vi "Arduino_Timed_Gate.vi"() -> (5 "Plug in titles":string[](array[string]), 7 "Plug in values":string[](array[string]))   [LabVIEW 2013]
uses:
  Controls/Post_Process.ctl
  Controls/Setup.ctl
  Globals/Meas_global.vi
panel:
  out "Current state":string
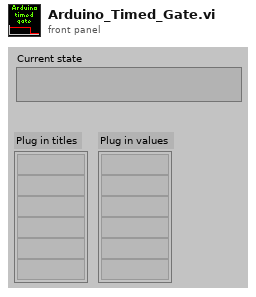
[diagram p1: front panel]
types:
  T1 = typedef "Setup.ctl" = enum16{"Run Program", "Show Setup", "Save Current Setup", "Setup Front Panel"}
  T2 = typedef "Post_Process.ctl" = enum16{"Take New Data", "Post Process Raw Data File"}
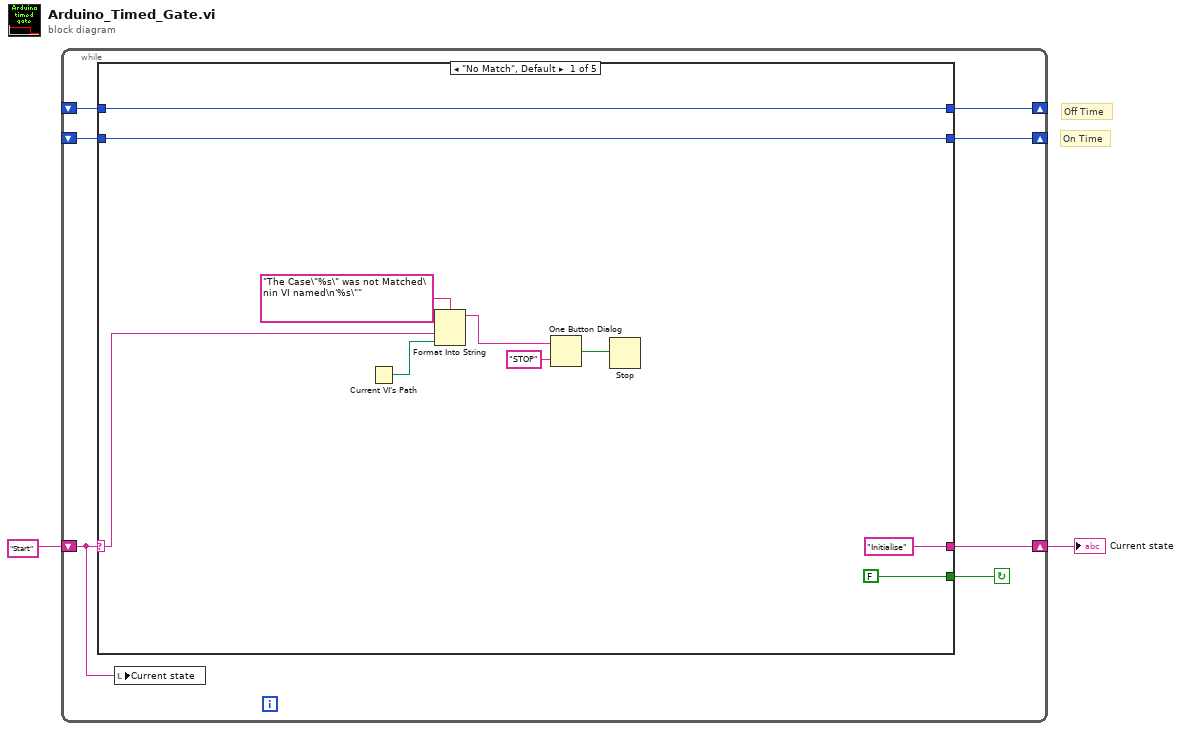
[diagram p0: block diagram]
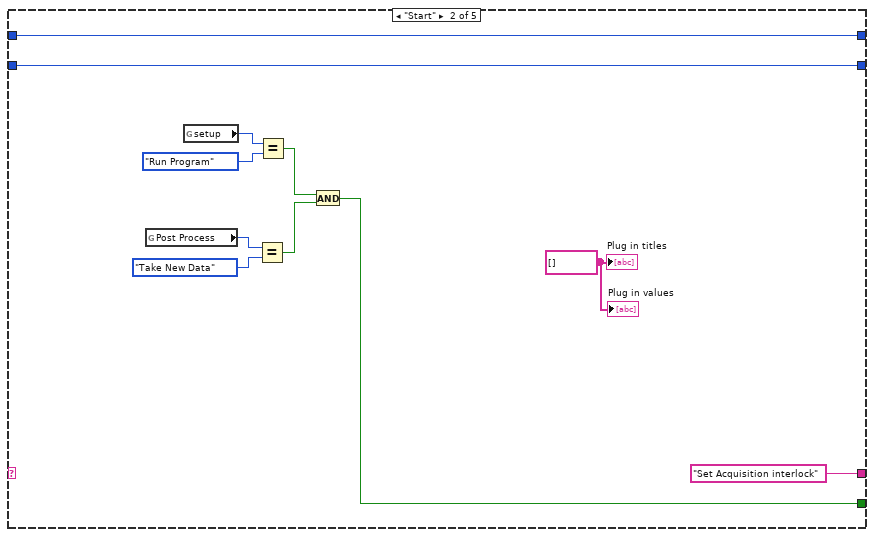
[diagram p2: hidden frame]
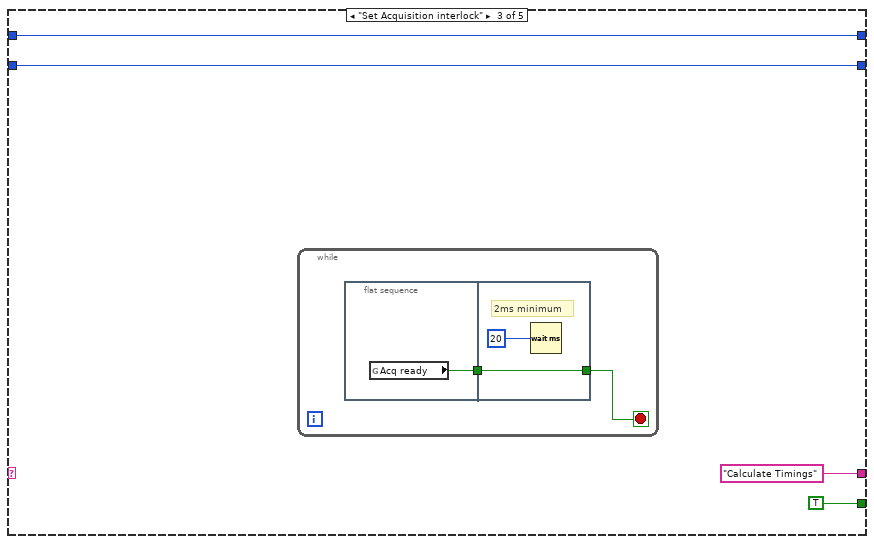
[diagram p3: hidden frame]
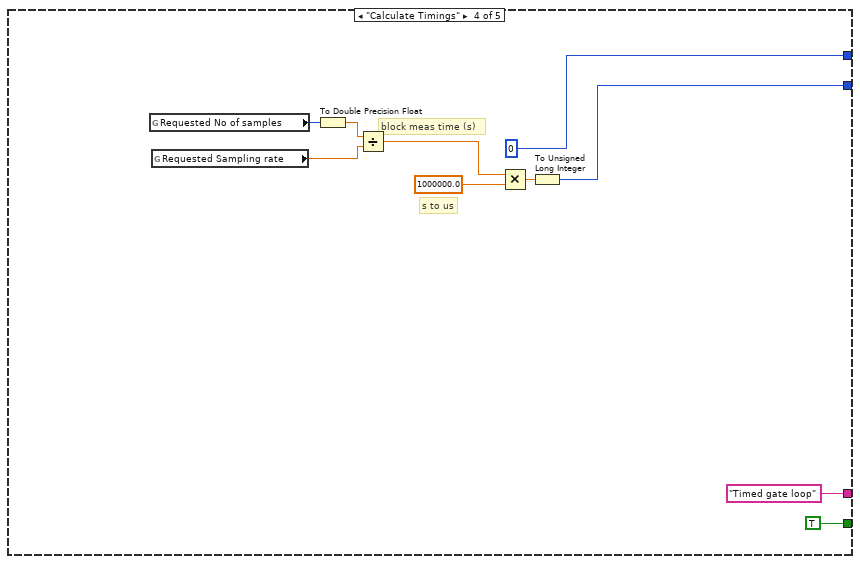
[diagram p4: hidden frame]
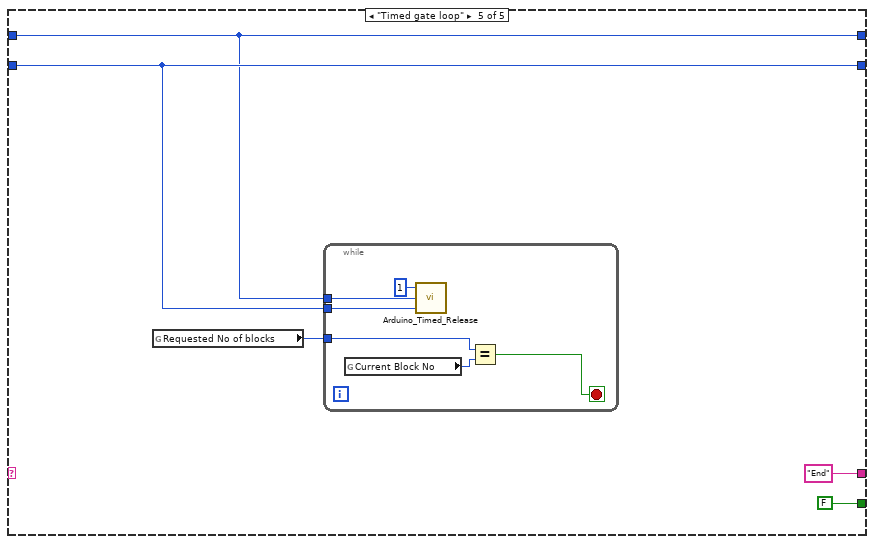
[diagram p5: hidden frame]
diagram:
  # "On Time"
  # "Off Time"
  n1 = while {
    shift-left: "Start" -> [w3]
    shift-right: [w8] -> w1
    shift-right: [w7] -> _
    shift-left: _ -> [w6]
    shift-right: [w5] -> _
    shift-left: _ -> [w4]
    stop <- w9 continue-if-true
    n2 = case shown="\"No Match\", Default" w3 {
      selector: w3 -> [w10 _ _ _ _]
      tunnel: [FALSE w22 TRUE ("Command Found") TRUE ("Command Found") FALSE ("Command Found")] -> w9
      tunnel: ["Initialise" "Set Acquisition interlock" "Calculate Timings" "Timed gate loop" "End"] -> w8
      tunnel: [w12 w21 w32 u32 0 ("number") w51] -> w7
      tunnel: w6 -> [w12 w21 w32 _ w51]
      tunnel: [w11 w20 w31 w44 w54] -> w5
      tunnel: w4 -> [w11 w20 w31 _ w54]
      frame "No Match", Default {
        n3 = Current VI's Path() -> (path=w14:path)
        n4 = Format Into String(format string="The Case\"%s\" was not Matched\nin VI named\n'%s\"" ("Format String"), w10, w14) -> (resulting string=w17:string)  [unwired: 2 in, 1 out]
        n5 = One Button Dialog(message=w17, button name ("OK")="STOP") -> (true=w15:bool)
        n6 = Stop(stop? (T)=w15) -> ()
      }
      frame "Start" {
        w29 = string[] [] ("Plug in titles")
        n7 = global read "Meas_global.vi" "Post Process"() -> (w24:T2)
        n8 = global read "Meas_global.vi" "setup"() -> (w23:T1)
        n9 = Equal?(x=w24, y=Post_Process."Take New Data" ("Post Process")) -> (x = y?=w27:bool)
        n10 = Equal?(x=w23, y=Setup."Run Program") -> (x = y?=w28:bool)
        n11 = And(x=w28, y=w27) -> (x .and. y?=w22:bool)
        "Plug in values" <- w29
        "Plug in titles" <- w29
      }
      frame "Set Acquisition interlock" {
        n12 = while {
          stop <- w36 stop-if-true
          n13 = flat-sequence {
            tunnel: [w37] -> w35
            tunnel: [w39] -> w36
            tunnel: w35 -> [w39]
            frame #0 {
              n14 = global read "Meas_global.vi" "Acq ready"() -> (w37:bool)
            }
            frame #1 {
              # "2ms minimum"
              n15 = Wait (ms)(milliseconds to wait=u32 20) -> ()  [unwired: 1 out]
            }
          }
        }
      }
      frame "Calculate Timings" {
        # "s to us"
        # "block meas time (s)"
        n16 = global read "Meas_global.vi" "Requested No of samples"() -> (w47:i32)
        n17 = global read "Meas_global.vi" "Requested Sampling rate"() -> (w45:dbl)
        n18 = To Double Precision Float(number=w47) -> (double precision float=w43:dbl)
        n19 = Divide(x=w43, y=w45) -> (x/y=w42:dbl)
        n20 = Multiply(x=w42, y=1000000.0) -> (x*y=w46:dbl)
        n21 = To Unsigned Long Integer(number=w46) -> (unsigned 32bit integer=w44:u32)
      }
      frame "Timed gate loop" {
        n22 = global read "Meas_global.vi" "Requested No of blocks"() -> (w50:i32)
        n23 = while {
          tunnel: w54 -> [w60]
          tunnel: w51 -> [w59]
          tunnel: w50 -> [w56]
          stop <- w55 stop-if-true
          n24 = global read "Meas_global.vi" "Current Block No"() -> (w57:i32)
          n25 = call "Arduino_Timed_Release.vi"("Time to hold source ON (microseconds)"=w60, "Time to hold source OFF (microseconds)"=w59, "Number of cycles"=u16 1) -> ()  [unwired: 2 out]
          n26 = Equal?(x=w56, y=w57) -> (x = y?=w55:bool)
        }
      }
    }
    n27 = local write "Current state"(w3) -> ()
  }
  "Current state" <- w1
